vi "GetImageReference.vi"(8 "error in (no error)":errorcluster, 10 "Image Name":string, 11 "GFG_Core VI Refnum IN":refnum<vi>) -> (0 "error out":errorcluster, 1 "Found?":bool, 2 "Image Reference out":T1, 3 "GFG_Core VI Refnum OUT":refnum<vi>)   [LabVIEW 2012]
doc: "SciScan 1.2 160622"
uses:
  <vilib>/vision/Image Controls.llb/IMAQ Image.ctl
panel:
  out "output cluster":T2
  out "Variant Out":variant
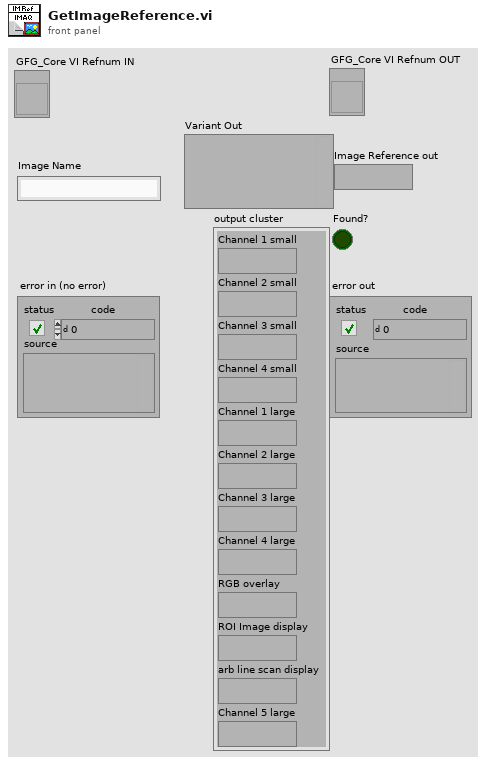
[diagram p1: front panel]
types:
  T1 = typedef "IMAQ Image.ctl" = refnum<image>
  T2 = cluster{"Channel 1 small":T1, "Channel 2 small":T1, "Channel 3 small":T1, "Channel 4 small":T1, "Channel 1 large":T1, "Channel 2 large":T1, "Channel 3 large":T1, "Channel 4 large":T1, "RGB overlay":T1, "ROI Image display":T1, "arb line scan display":T1, "Channel 5 large":T1}
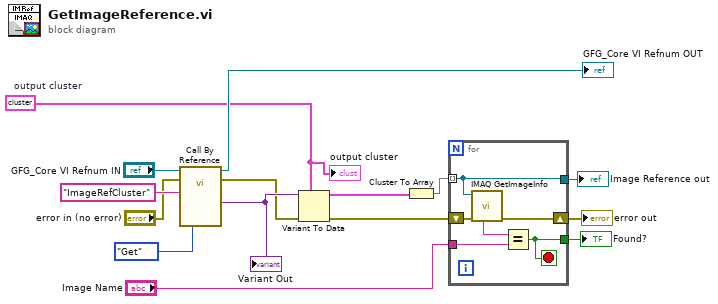
[diagram p0: block diagram]
diagram:
  w3 = T2 {"Channel 1 small"=refnum, "Channel 2 small"=refnum, "Channel 3 small"=refnum, "Channel 4 small"=refnum, "Channel 1 large"=refnum, "Channel 2 large"=refnum, "Channel 3 large"=refnum, "Channel 4 large"=refnum, "RGB overlay"=refnum, "ROI Image display"=refnum, "arb line scan display"=refnum, "Channel 5 large"=refnum}  # output cluster
  n1 = call-by-ref "?"(reference="GFG_Core VI Refnum IN", error in="error in (no error)", "Variable Name in"="ImageRefCluster", "Action"=enum16{"Init", "Set", "Get"}."Get") -> (reference out=→"GFG_Core VI Refnum OUT":refnum<vi>, error out=w1:errorcluster, "Variant Out"=w12:variant)  [unwired: 11 in, 6 out]
  "Variant Out" <- w12
  n2 = Variant To Data(error in=w1, type=w3, Variant=w12) -> (data=w11:T2, error out=w6:errorcluster)
  n3 = Cluster To Array(cluster=w11) -> (array=w10:T1[])
  n4 = for {
    tunnel: w10 -> [w18] mode=indexing
    tunnel: "Image Name" -> [w20]
    tunnel: [w19] -> w8
    tunnel: [w18] -> w7
    shift-right: [w16] -> w5
    shift-left: w6 -> [w17]
    stop <- w19 stop-if-true
    n5 = call "IMAQ GetImageInfo"("error in (no error)"=w17, "Image"=w18) -> ("error out"=w16:errorcluster, "Image Name"=w21:string)  [unwired: 2 in, 6 out]
    n6 = Equal?(x=w21, y=w20) -> (x = y?=w19:bool)
  }
  "error out" <- w5
  "Found?" <- w8
  "Image Reference out" <- w7
  "output cluster" <- w3
